vi "Part 1.vi"(11 "Input":string) -> (3 "Output":i64)   [LabVIEW 2021]
uses:
  66d7226d-6358-4fb9-ab82-74928c424c26.vi
  <userlib>/_OpenG.lib/string/string.llb/Convert EOLs (String)__ogtk.vi
  <vilib>/Comparison/Less/Less Functor/Less Functor.lvclass
panel:
  out "Monkeys":T1(array[cluster])
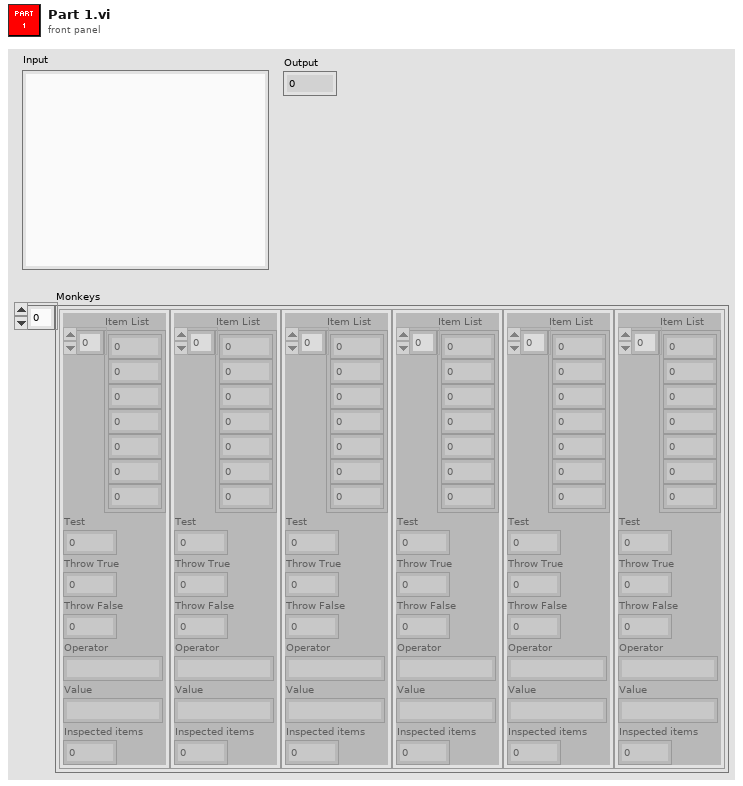
[diagram p1: front panel]
types:
  T1 = cluster{"Item List":i64[], "Test":i64, "Throw True":i64, "Throw False":i64, "Operator":string, "Value":string, "Inspected items":i64}[]
  T2 = cluster{"Item List":i64[], "Test":i64, "Throw True":i64, "Throw False":i64, "Operator":string, "Value":string, "Inspected items":i64}
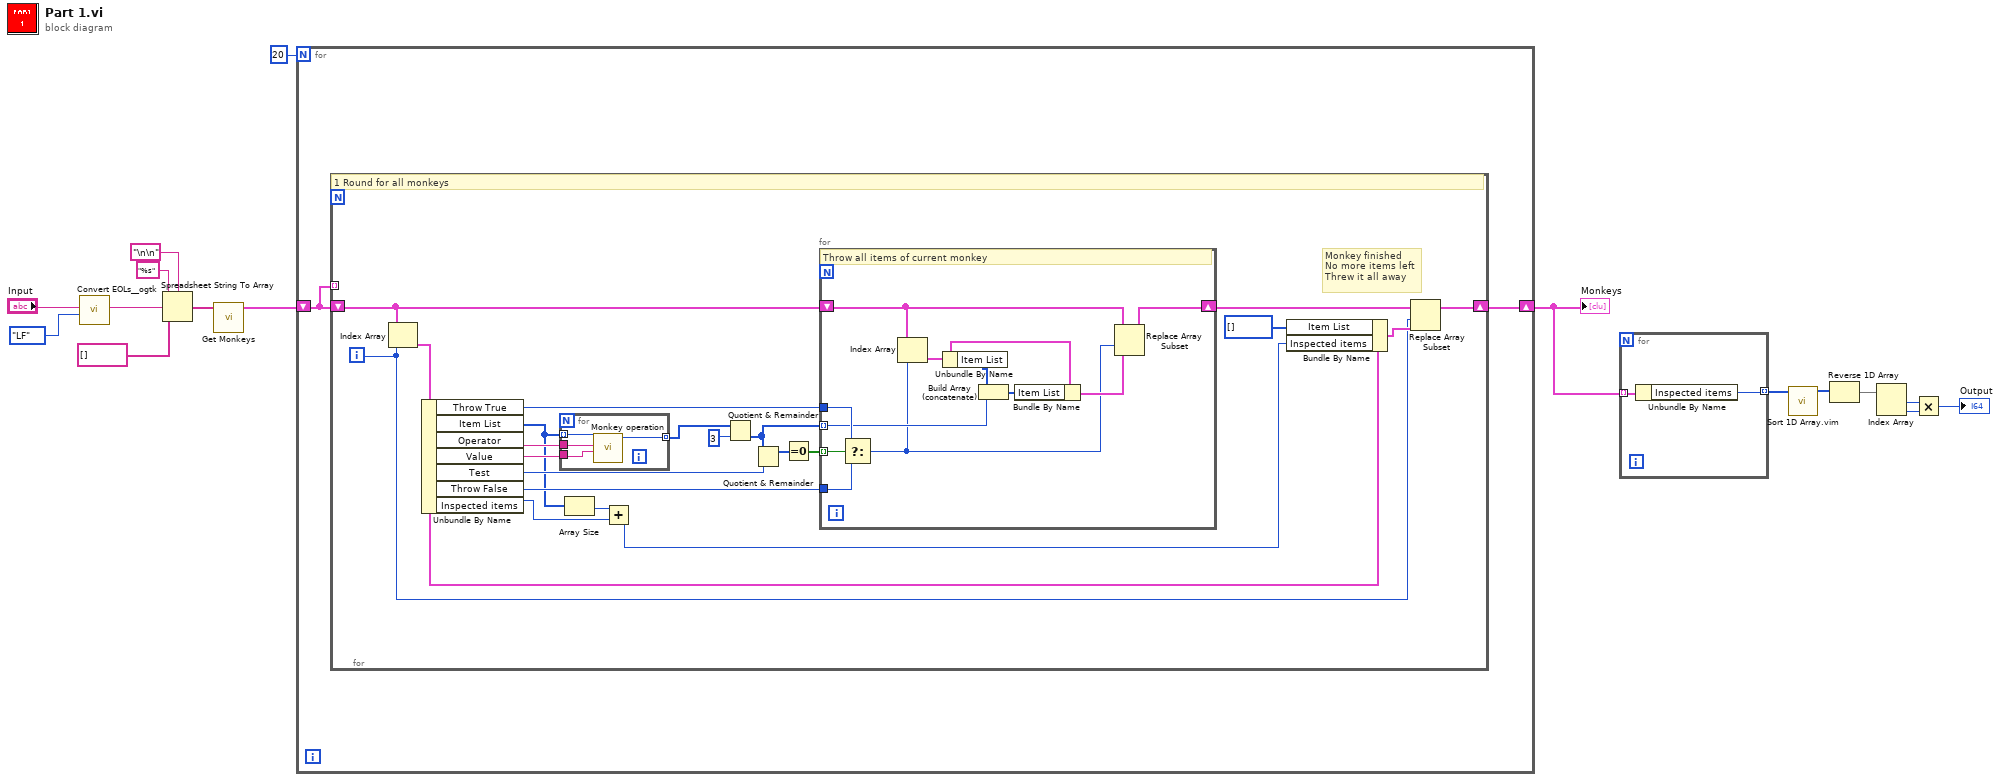
[diagram p0: block diagram]
diagram:
  n1 = call-poly <userlib>:"Convert EOLs__ogtk.vi"("Convert to:"=enum16{"CR", "LF", "CRLF"}."LF", "String in"="Input") -> ("String out"=w14:string)  [unwired: 9 in]
  n2 = Spreadsheet String To Array(delimiter (Tab)="\n\n", format string="%s", spreadsheet string=w14, array type (2D Dbl)=string[] []) -> (array=w12:string[])
  n3 = call "Get Monkeys.vi"("Array in"=w12) -> ("Monkeys"=w9:T1)  [unwired: 9 in, 1 out]
  n4 = for {
    N: 20 -> [_]
    shift-right: [w17] -> w7
    shift-left: w9 -> [w18]
    n5 = for {
      shift-right: [w38] -> w17
      shift-left: w18 -> [w32]
      tunnel: w18 -> [_] mode=indexing
      i -> [w29]
      # "Monkey finished\nNo more items left\nThrew it all away"
      # "1 Round for all monkeys"
      n6 = Index Array(array=w32, index=w29) -> (element=w30:T2)
      n7 = Unbundle By Name(w30) -> ("Throw True"=w33:i64, "Item List"=w22:i64[], "Operator"=w25:string, "Value"=w24:string, "Test"=w26:i64, "Throw False"=w27:i64, "Inspected items"=w20:i64)
      n8 = for {
        tunnel: w25 -> [w43]
        tunnel: w24 -> [w42]
        tunnel: w22 -> [w41] mode=indexing
        tunnel: [w40] -> w23 mode=indexing
        n9 = call "Monkey operation.vi"("Value"=w42, "Operator"=w43, "Old"=w41) -> ("New"=w40:i64)  [unwired: 8 in]
      }
      n10 = Array Size(array=w22) -> (size(s)=w21:i32)
      n11 = Add(x=w21, y=w20) -> (x+y=w19:i64)
      n12 = Quotient & Remainder(x=w23, y=i64 3) -> (floor(x/y)=w28:i64[])  [unwired: 1 out]
      n13 = Quotient & Remainder(x=w28, y=w26) -> (x-y*floor(x/y)=w35:i64[])  [unwired: 1 out]
      n14 = Equal To 0?(x=w35) -> (x = 0?=w34:bool[])
      n15 = for {
        tunnel: w34 -> [w54] mode=indexing
        tunnel: w33 -> [w53]
        tunnel: w27 -> [w52]
        shift-right: [w44] -> w31
        shift-left: w32 -> [w45]
        tunnel: w28 -> [w50] mode=indexing
        # "Throw all items of current monkey"
        n16 = Select(t=w53, s=w54, f=w52) -> (s? t:f=w46:i64)
        n17 = Index Array(array=w45, index=w46) -> (element=w49:T2)
        n18 = Unbundle By Name(w49) -> ("Item List"=w51:i64[])
        n19 = Build Array (concatenate)(w51, w50) -> (w48:i64[])
        n20 = Bundle By Name(cluster=w49, "Item List"=w48) -> (w47:T2)
        n21 = Replace Array Subset(array=w45, new element=w47, index=w46) -> (w44:T1)
      }
      n22 = Bundle By Name(cluster=w30, "Item List"=i64[] [], "Inspected items"=w19) -> (w37:T2)
      n23 = Replace Array Subset(array=w31, new element=w37, index=w29) -> (w38:T1)
    }
  }
  "Monkeys" <- w7
  n24 = for {
    tunnel: w7 -> [w56] mode=indexing
    tunnel: [w55] -> w6 mode=indexing
    n25 = Unbundle By Name(w56) -> ("Inspected items"=w55:i64)
  }
  n26 = call "Sort 1D Array.vim"("unsorted array"=w6) -> ("sorted array"=w5:i64[])  [unwired: 10 in]
  n27 = Reverse 1D Array(array=w5) -> (reversed array=w4:i64[])
  n28 = Index Array(array=w4) -> (element #1=w3:i64, element #2=w2:i64)  [unwired: 2 in]
  n29 = Multiply(x=w3, y=w2) -> (x*y=→"Output":i64)
